vi "ball speed.vi"(8 "Falling Edge":bool, 9 "Rising Edge":bool, 11 "Distance (in)":dbl) -> (3 "speed (ft/s)":dbl)   [LabVIEW 2011]
uses:
  <vilib>/Rock Robotics/WPI/Counter/WPI_CounterDigitalInputToDigitalSource.vi
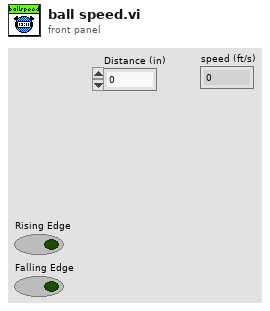
[diagram p1: front panel]
types:
  T1 = typedef "WPI_DigitalInputDevRef.ctl" = cluster{"DevStatus":errorcluster, "DIO Channel":T2, "Digital Module":T3}
  T2 = typedef "FPGA_DIOChannel.ctl" = enum8{"DIO 1", "DIO 2", "DIO 3", "DIO 4", "DIO 5", "DIO 6", "DIO 7", "DIO 8", "DIO 9", "DIO 10", "DIO 11", "DIO 12", "DIO 13", "DIO 14", "Invalid"}
  T3 = typedef "FPGA_TypedefDigitalModule.ctl" = enum16{"Digital Module 1", "Digital Module 2"}
  T4 = typedef "FPGA_CounterEncoderSourceConvertionLVSourceType.ctl" = cluster{"DevStatus":errorcluster, "AnalogTriggerMode?":bool, "DigitalMode":cluster{"Digital Module":T3, "DIO Channel":T5}, "AnalogTriggerMode":cluster{"AnalogTriggerIndex":T6, "OutputType":T7}}
  T5 = typedef "FPGA_DIODigitalSourceChannel.ctl" = enum8{"DIO 1", "DIO 2", "DIO 3", "DIO 4", "DIO 5", "DIO 6", "DIO 7", "DIO 8", "DIO 9", "DIO 10", "DIO 11", "DIO 12", "DIO 13", "DIO 14", "Disabled"}
  T6 = typedef "FPGA_AnalogTriggerIndex.ctl" = enum8{"Trig 0", "Trig 1", "Trig 2", "Trig 3", "Trig 4", "Trig 5", "Trig 6", "Trig 7", "Invalid"}
  T7 = typedef "FPGA_AnalogTriggerOutType.ctl" = enum16{"InWindow", "TriggerState", "Rising", "Falling"}
  T8 = typedef "WPI_InterruptRef.ctl" = cluster{"DevStatus":errorcluster, "InterruptIndex":T9}
  T9 = typedef "FPGA_InterruptIndex.ctl" = enum8{"0", "1", "2", "3", "4", "5", "6", "7", "Invalid"}
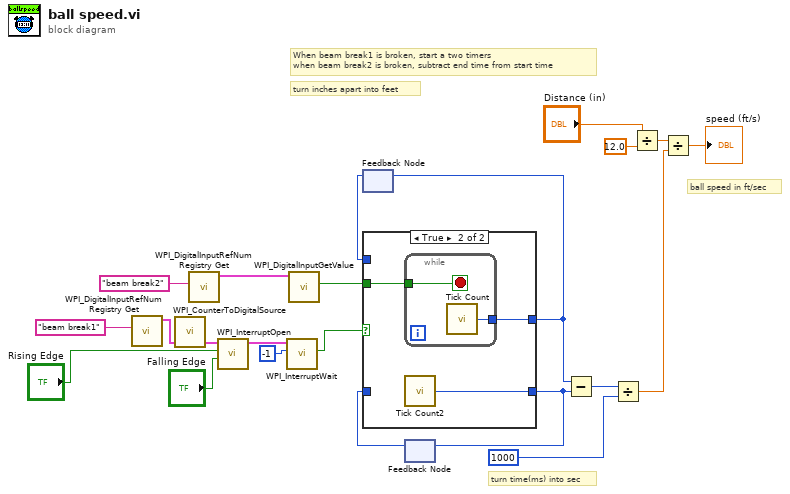
[diagram p0: block diagram]
diagram:
  # "ball speed in ft/sec"
  # "turn time(ms) into sec"
  # "turn inches apart into feet"
  # "When beam break1 is broken, start a two timers\nwhen beam break2 is broken, subtract end time from start time"
  n1 = call <vilib>:"WPI_DigitalInputRefNum Registry Get.vi"("refnum name"="beam break1") -> ("DigitalInputDevRef"=w7:T1)  [unwired: 9 in, 1 out]
  n2 = call-poly <vilib>:"WPI_CounterToDigitalSource.vi"("DigitalInputDevRef"=w7) -> ("Digital Source"=w6:T4)  [unwired: 6 in]
  n3 = call <vilib>:"WPI_DigitalInputRefNum Registry Get.vi"("refnum name"="beam break2") -> ("DigitalInputDevRef"=w20:T1)  [unwired: 9 in, 1 out]
  n4 = call <vilib>:"WPI_InterruptOpen.vi"("Falling Edge"="Falling Edge", "Rising Edge"="Rising Edge", "Source"=w6) -> ("InterruptRef"=w3:T8)  [unwired: 7 in, 1 out]
  n5 = call <vilib>:"WPI_InterruptWait.vi"("Timeout (ms)"=-1, "InterruptRef"=w3) -> ("Timed Out"=w1:bool)  [unwired: 6 in, 3 out]
  n6 = call <vilib>:"WPI_DigitalInputGetValue.vi"("DigitalInputDevRef"=w20) -> ("Value"=w17:bool)  [unwired: 8 in, 2 out]
  n7 = feedback #1() -> (w19:u32)  [unwired: 1 in]
  n8 = feedback #2() -> (w18:u32)  [unwired: 1 in]
  n9 = case shown="True" w1 {
    tunnel: [w23 w27] -> w15
    tunnel: [w24 w26] -> w16
    tunnel: w19 -> [w24 _]
    tunnel: w18 -> [w23 _]
    tunnel: w17 -> [_ w25]
    frame False {
    }
    frame True {
      n10 = while {
        tunnel: [w29] -> w26
        tunnel: w25 -> [w28]
        stop <- w28 stop-if-true
        n11 = call "Tick Count"() -> ("Tick Count(mSec)"=w29:u32)
      }
      n12 = call "Tick Count2"() -> ("Tick Count(mSec)"=w27:u32)
    }
  }
  n13 = feedback-in #1(w16) -> ()
  n14 = feedback-in #2(w15) -> ()
  n15 = Subtract(x=w16, y=w15) -> (x-y=w12:u32)
  n16 = Divide(x=w12, y=u32 1000) -> (x/y=w10:dbl)
  n17 = Divide(x="Distance (in)", y=12.0) -> (x/y=w9:dbl)
  n18 = Divide(x=w9, y=w10) -> (x/y=→"speed (ft/s)":dbl)
